vi "Set from JSON string.vi"(8 "error in (no error)":errorcluster, 10 "JSON stream":string, 11 "JSON Value in":refnum<class "JSON Value.lvclass">) -> (0 "error out":errorcluster, 2 "rest of JSON stream":string, 3 "JSON Value out":refnum<class "JSON Value.lvclass">)   [LabVIEW 2020, in "Library Commun.lvlib" / "JSON Value.lvclass"]
doc: "Converts a <b>JSON stream</b> into a <b>JSON Value</b>.\n\nCopyright 2012 James David Powell, Shaun Rumbell and Ton Plomp\nMore information on http://lavag.org/topic/16217-cr-json-labview"
uses:
  JSON Value.lvclass
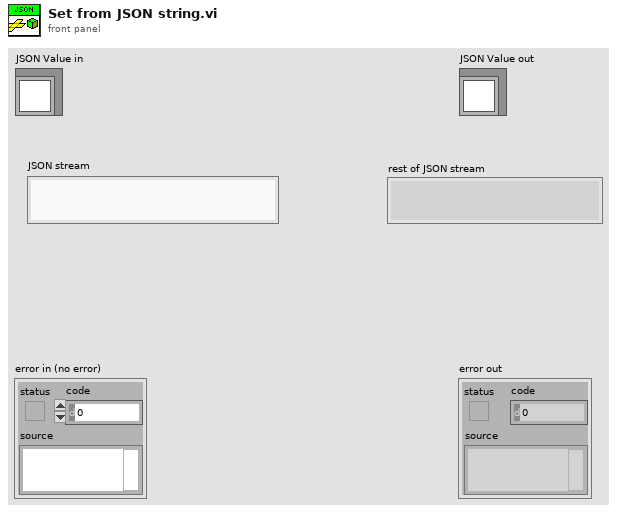
[diagram p1: front panel]
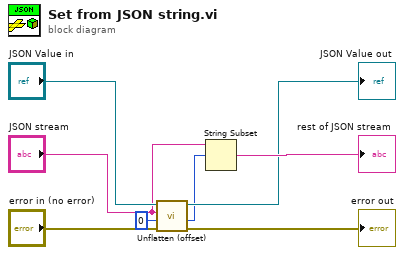
[diagram p0: block diagram]
diagram:
  n1 = call-dynamic "Unflatten (offset).vi"("error in (no error)"="error in (no error)", "offset (0)"=0, "JSON stream"="JSON stream", "JSON Value in"="JSON Value in") -> ("error out"=→"error out":errorcluster, "offset"=w1:i32, "JSON Value out"=→"JSON Value out":refnum<class "JSON Value.lvclass">)  [unwired: 4 in, 1 out]
  n2 = String Subset(string="JSON stream", offset (0)=w1) -> (substring=→"rest of JSON stream":string)  [unwired: 1 in]
